vi "dfd_Cosine-Modulated Prototype Filter Param Validation.vi"(4 "PR?":u16(ring) items=["NPR", "PR"], 6 "weight":dbl=0.5, 7 "number of bands":i32=4, 8 "error in (no error)":errorcluster, 10 "roll off":dbl=0.2, 11 "order":i32=38) -> (0 "error out":errorcluster, 2 "dup roll off":dbl, 3 "dup order":i32)   [LabVIEW 2017, in "NI_DigFilter_FilterBank.lvlib"]
doc: "Validates the parameters for the prototype filter design. If any parameter is not in their range, this VI will give an error report. If the order is not an integer of 2kM this VI will give a warning report, where k is any positive integer, and M is specified by <B>number of bands</B>."
uses:
  <vilib>/addons/Digital Filter Design/NI_DigFilter_FilterBank.lvlib
  <vilib>/addons/Digital Filter Design/_Misc.llb/dfd_Error Handlers (Multiple).vi
  <vilib>/addons/Digital Filter Design/NI_DigFilterLicensed.lvlib
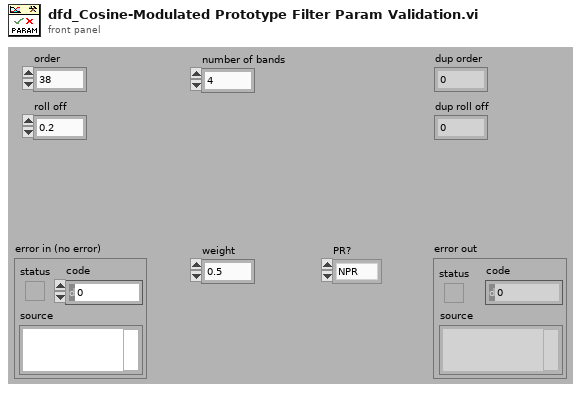
[diagram p1: front panel]
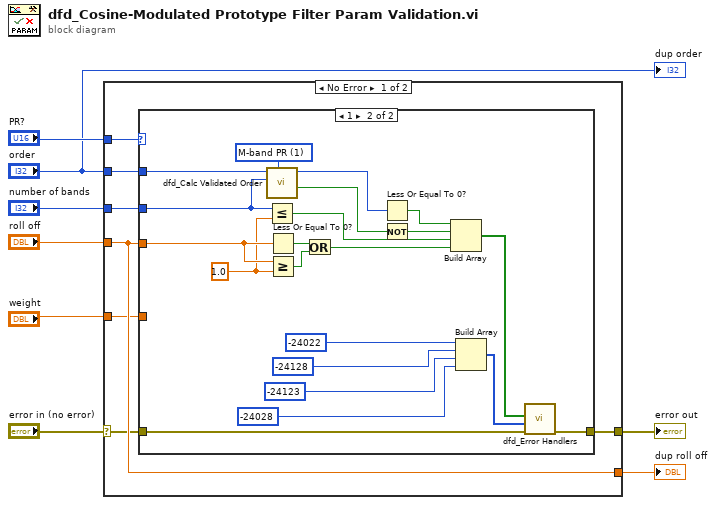
[diagram p0: block diagram]
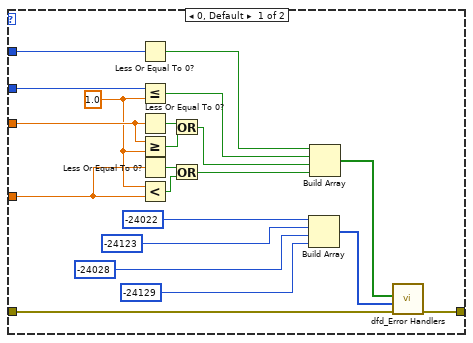
[diagram p2: hidden frame]
diagram:
  n1 = case shown="No Error" "error in (no error)" {
    selector: "error in (no error)" -> [w12 w58]
    tunnel: "order" -> [w10 _]
    tunnel: "roll off" -> [w14 _]
    tunnel: "weight" -> [w13 _]
    tunnel: "number of bands" -> [w11 _]
    tunnel: [w15 w58] -> w5
    tunnel: [w14 _] -> w3
    tunnel: "PR?" -> [w9 _]
    frame No Error {
      n2 = case shown="1" w9 {
        tunnel: [w34 w55] -> w15
        tunnel: w14 -> [w32 w53]
        tunnel: w13 -> [w20 _]
        tunnel: w12 -> [w29 w50]
        tunnel: w11 -> [w16 w41]
        tunnel: w10 -> [w17 w42]
        frame 0, Default {
          w21 = 1.0
          n3 = Less Or Equal To 0?(x=w17) -> (x <= 0?=w18:bool)
          n4 = Less Or Equal?(x=w16, y=w21) -> (x <= y?=w26:bool)
          n5 = Less Or Equal To 0?(x=w32) -> (x <= 0?=w33:bool)
          n6 = Greater Or Equal?(x=w32, y=w21) -> (x >= y?=w31:bool)
          n7 = Less Or Equal To 0?(x=w20) -> (x <= 0?=w22:bool)
          n8 = Less?(x=w21, y=w20) -> (x < y?=w23:bool)
          n9 = Or(x=w33, y=w31) -> (x .or. y?=w30:bool)
          n10 = Or(x=w22, y=w23) -> (x .or. y?=w19:bool)
          n11 = Build Array(-24022 ("ERR_ORDER_LE_ZERO"), -24123 ("ERR_INVALID_BAND_NUM"), -24028 ("ERR_ROLLOFF_RANGE_WRONG"), -24129 ("ERR_INVALID_WEIGHT")) -> (w35:i32[])
          n12 = Build Array(w18, w26, w30, w19) -> (w36:bool[])
          n13 = call-poly <vilib>:"dfd_Error Handlers.vi"("error in (no error)"=w29, "error sources"=w35, "condition failed?"=w36) -> ("error out"=w34:errorcluster)  [unwired: 8 in]
        }
        frame 1 {
          w40 = u16 1 items=["2-band", "M-band PR"] ("bank type")
          w48 = 1.0
          n14 = call <vilib>:"dfd_Calc Validated Order.vi"("bank type"=w40, "bank counts"=w41, "order"=w42) -> ("valid?"=w38:bool, "dup order"=w37:i32)  [unwired: 6 in, 1 out]
          n15 = Less Or Equal?(x=w41, y=w48) -> (x <= y?=w45:bool)
          n16 = Less Or Equal To 0?(x=w53) -> (x <= 0?=w54:bool)
          n17 = Greater Or Equal?(x=w53, y=w48) -> (x >= y?=w52:bool)
          n18 = Or(x=w54, y=w52) -> (x .or. y?=w51:bool)
          n19 = Less Or Equal To 0?(x=w37) -> (x <= 0?=w44:bool)
          n20 = Not(x=w38) -> (.not. x?=w39:bool)
          n21 = Build Array(w44, w39, w45, w51) -> (w57:bool[])
          n22 = Build Array(-24022 ("ERR_ORDER_LE_ZERO"), -24128 ("ERR_ORDER_PR_MBAND"), -24123 ("ERR_INVALID_BAND_NUM"), -24028 ("ERR_ROLLOFF_RANGE_WRONG")) -> (w56:i32[])
          n23 = call-poly <vilib>:"dfd_Error Handlers.vi"("error in (no error)"=w50, "error sources"=w56, "condition failed?"=w57) -> ("error out"=w55:errorcluster)  [unwired: 8 in]
        }
      }
    }
    frame Error {
    }
  }
  "error out" <- w5
  "dup roll off" <- w3
  "dup order" <- "order"
